vi "Calculate Channel Value.vi"(8 "error in (no error)":errorcluster, 9 "Digital":bool=TRUE, 10 "Step Settings":T1, 11 "Output Sequencer in":refnum<class "Output Sequencer.lvclass">) -> (0 "error out":errorcluster, 2 "Values to Write":dbl[](array[numeric]), 3 "Output Sequencer out":refnum<class "Output Sequencer.lvclass">)   [LabVIEW 2020, in "Output Sequencer.lvlib" / "Output Sequencer.lvclass"]
uses:
  Output Sequencer.lvclass
  Types/Compiled Step.ctl
  <vilib>/LAVA/muParser/mupExpr/mupExpr.lvclass
  Types/Expression Data.ctl
  Output Sequencer.lvclass/Output Sequencer.ctl
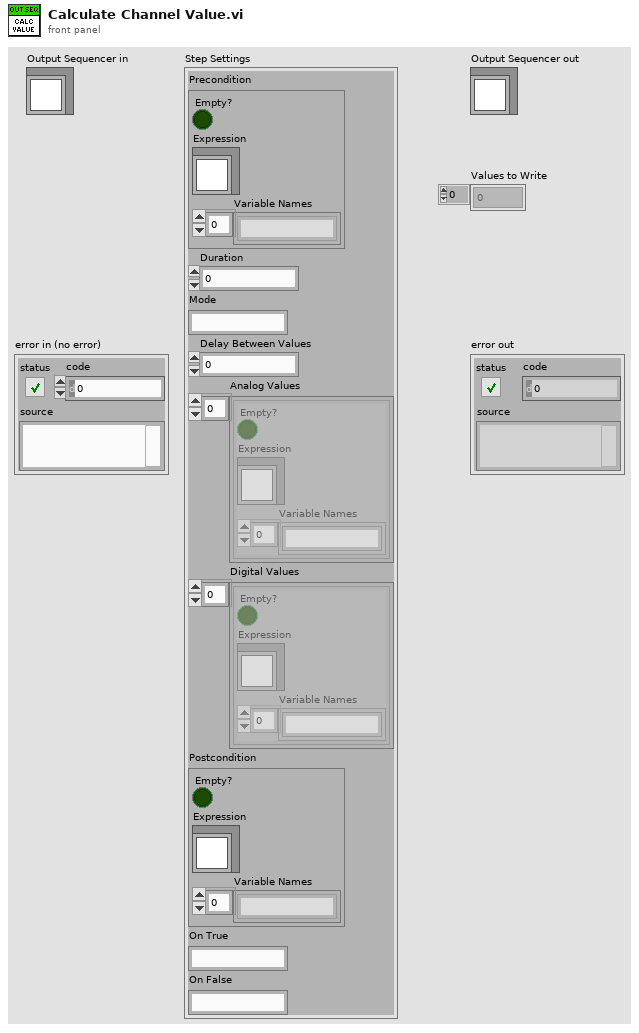
[diagram p1: front panel]
types:
  T1 = typedef "Output Sequencer.lvlib/Output Sequencer.lvclass/Compiled Step.ctl" = cluster{"Precondition":T2, "Duration":dbl, "Mode":string, "Delay Between Values":dbl, "Analog Values":T2[], "Digital Values":T2[], "Postcondition":T2, "On True":string, "On False":string}
  T2 = typedef "Output Sequencer.lvlib/Output Sequencer.lvclass/Expression Data.ctl" = cluster{"Empty?":bool, "Expression":refnum<class "mupExpr.lvclass">, "Variable Names":string[]}
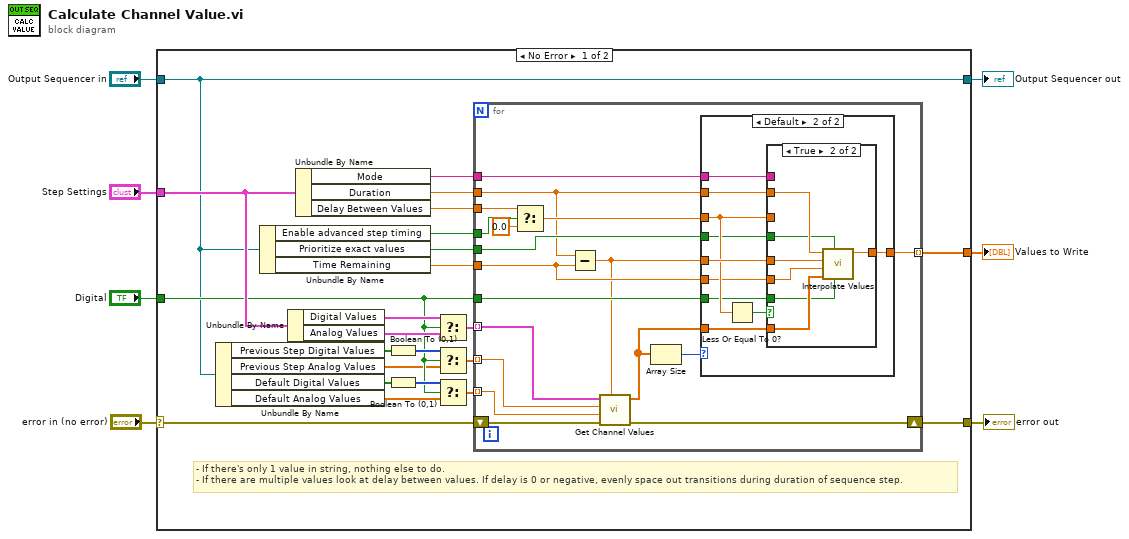
[diagram p0: block diagram]
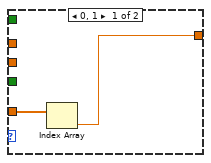
[diagram p2: hidden frame]
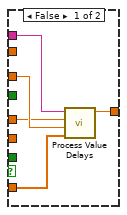
[diagram p3: hidden frame]
diagram:
  n1 = case shown="No Error" "error in (no error)" {
    selector: "error in (no error)" -> [w8 w73]
    tunnel: "Step Settings" -> [w30 _]
    tunnel: [w27 _] -> w6
    tunnel: "Digital" -> [w20 _]
    tunnel: "Output Sequencer in" -> [w9 w74]
    tunnel: [w15 w73] -> w3
    tunnel: [w9 w74] -> w2
    frame No Error {
      # "- If there's only 1 value in string, nothing else to do. \n- If there are multiple values look at delay between values. If delay is 0 or negative, evenly space out transitions during duration of sequence step."
      n2 = Unbundle By Name(w9) -> ("Previous Step Digital Values"=w17:bool[], "Previous Step Analog Values"=w18:dbl[], "Default Digital Values"=w21:bool[], "Default Analog Values"=w23:dbl[])
      n3 = Unbundle By Name(w9) -> ("Enable advanced step timing"=w13:bool, "Prioritize exact values"=w14:bool, "Time Remaining"=w16:dbl)
      n4 = Unbundle By Name(w30) -> ("Digital Values"=w29:T2[], "Analog Values"=w28:T2[])
      n5 = Unbundle By Name(w30) -> ("Mode"=w12:string, "Duration"=w11:dbl, "Delay Between Values"=w10:dbl)
      n6 = Boolean To (0,1)(Boolean=w17) -> (0, 1=w24:i16[])
      n7 = Boolean To (0,1)(Boolean=w21) -> (0, 1=w22:i16[])
      n8 = Select(t=w29, s=w20, f=w28) -> (s? t:f=w26:T2[])
      n9 = Select(t=w24, s=w20, f=w18) -> (s? t:f=w25:dbl[])
      n10 = Select(t=w22, s=w20, f=w23) -> (s? t:f=w19:dbl[])
      n11 = for {
        tunnel: w26 -> [w43] mode=indexing
        tunnel: w20 -> [w46]
        tunnel: w16 -> [w45]
        tunnel: [w44] -> w27 mode=indexing
        tunnel: w25 -> [w42] mode=indexing
        tunnel: w19 -> [w41] mode=indexing
        tunnel: w14 -> [w40]
        tunnel: w13 -> [w39]
        shift-right: [w34] -> w15
        shift-left: w8 -> [w35]
        tunnel: w12 -> [w33]
        tunnel: w11 -> [w32]
        tunnel: w10 -> [w31]
        n12 = Select(t=w31, s=w39, f=0.0) -> (s? t:f=w37:dbl)
        n13 = Subtract(x=w32, y=w45) -> (x-y=w36:dbl)
        n14 = call "Get Channel Values.vi"("Time in Step"=w36, "error in (no error)"=w35, "Default Value"=w41, "Previous Value"=w42, "Channel Value Expression"=w43) -> ("error out"=w34:errorcluster, "Channel Values"=w47:dbl[])  [unwired: 5 in]
        n15 = Array Size(array=w47) -> (size(s)=w48:i32)
        n16 = case shown="Default" w48 {
          tunnel: w47 -> [w50 w59]
          tunnel: [w49 w55] -> w44
          tunnel: w37 -> [_ w57]
          tunnel: w36 -> [_ w58]
          tunnel: w33 -> [_ w56]
          tunnel: w32 -> [_ w54]
          tunnel: w46 -> [_ w53]
          tunnel: w45 -> [_ w52]
          tunnel: w40 -> [_ w51]
          frame 0, 1 {
            n17 = Index Array(array=w50) -> (element=w49:dbl)  [unwired: 1 in]
          }
          frame Default {
            n18 = Less Or Equal To 0?(x=w57) -> (x <= 0?=w60:bool)
            n19 = case shown="True" w60 {
              tunnel: w59 -> [w62 w68]
              tunnel: w58 -> [w63 w70]
              tunnel: w57 -> [w64 _]
              tunnel: w56 -> [w61 _]
              tunnel: [w65 w72] -> w55
              tunnel: w54 -> [_ w71]
              tunnel: w53 -> [_ w67]
              tunnel: w52 -> [_ w69]
              tunnel: w51 -> [_ w66]
              frame False {
                n20 = call "Process Value Delays.vi"("Values"=w62, "Delay"=w64, "Time in Step"=w63, "Mode"=w61) -> ("Value out"=w65:dbl)  [unwired: 7 in]
              }
              frame True {
                n21 = call "Interpolate Values.vi"("Digital"=w67, "Prioritize reaching values"=w66, "Values"=w68, "Remaining Time"=w69, "Time in Step"=w70, "Duration"=w71) -> ("Value Out"=w72:dbl)  [unwired: 5 in]
              }
            }
          }
        }
      }
    }
    frame Error {
    }
  }
  "Values to Write" <- w6
  "Output Sequencer out" <- w2
  "error out" <- w3
